vi "doFocus_max-xy.vi"(4 "WFChart Refnum":refnum<vi>, 6 "pixel_dwell_ms":dbl=0.1 caption="Dwell time ms:", 7 "pos_start":enum32{"bottom-left", "center"}(ring), 8 "frame_size_x_px":i32=50, 9 "image_size_x_um":dbl=6.0, 10 "pos-start_y":dbl=6.0, 11 "pos-start_x":dbl=6.0) -> (1 "focus_data":T1, 2 "z-focus":dbl)   [LabVIEW 2014]
panel:
  out "Intensity Graph":dbl[][](graph)
  # "Inputs"
  # "Outputs"
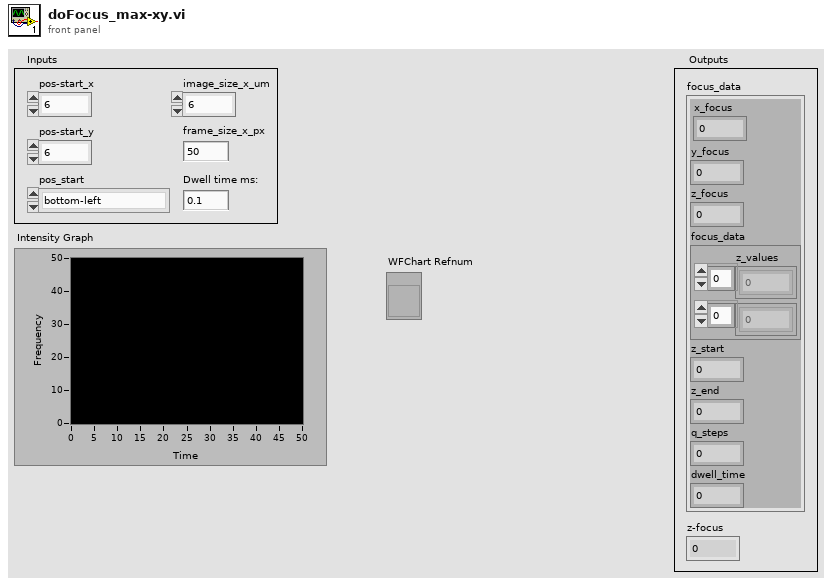
[diagram p1: front panel]
types:
  T1 = cluster{"x_focus":dbl, "y_focus":dbl, "z_focus":dbl, "focus_data":cluster{"z_values":dbl[], dbl[]}, "z_start":dbl, "z_end":dbl, "q_steps":i32, "dwell_time":dbl}
  T2 = cluster{dbl, dbl, "z_focus":dbl, "focus_data":cluster{"z_values":dbl[], dbl[]}, "z_start":dbl, "z_end":dbl, "q_steps":i32, "dwell_time":dbl}
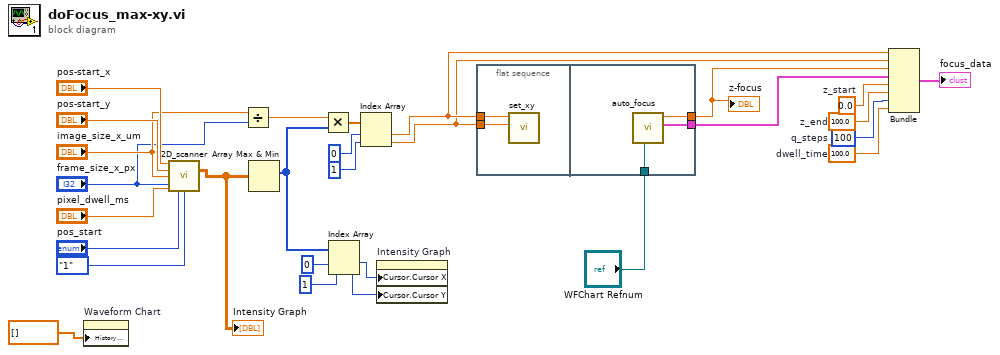
[diagram p0: block diagram]
diagram:
  w3 = 100.0  # dwell_time
  w4 = 100  # q_steps
  w5 = 100.0  # z_end
  w6 = 0.0  # z_start
  n1 = property on="Waveform Chart" class="WFChart (strict)"("History Data"=dbl[] []) -> ()  [unwired: 2 in, 2 out]
  n2 = call "2D_scanner.vi"("pos-start_x"="pos-start_x", "pos-start_y"="pos-start_y", "image_size_x_um"="image_size_x_um", "frame_size_x_px"="frame_size_x_px", "pixel_dwell_ms"="pixel_dwell_ms", "pos_start"="pos_start", "scan_direction"=enum32{"0", "1"}."1") -> ("image_out"=w17:dbl[][])  [unwired: 8 in]
  "Intensity Graph" <- w17
  n3 = Divide(x="image_size_x_um", y="frame_size_x_px") -> (x/y=w22:dbl)
  n4 = Array Max & Min(array=w17) -> (max index (indices)=w16:i32[])  [unwired: 3 out]
  n5 = Multiply(x=w22, y=w16) -> (x*y=w21:dbl[])
  n6 = Index Array(array=w16, index #1=0 ("index"), index #2=1 ("index")) -> (element #1=w13:i32, element #2=w12:i32)
  n7 = Index Array(array=w21, index #1=0 ("index"), index #2=1 ("index")) -> (element #1=w10:dbl, element #2=w9:dbl)
  n8 = property on="Intensity Graph" class="IntGraph (strict)"("Cursor.Cursor X"=w13, "Cursor.Cursor Y"=w12) -> ()  [unwired: 2 in, 2 out]
  n9 = flat-sequence {
    tunnel: w10 -> [w30]
    tunnel: w9 -> [w29]
    tunnel: "WFChart Refnum" -> [w33]
    tunnel: [w32] -> w8
    tunnel: [w31] -> w7
    frame #0 {
      n10 = call "set_xy.vi"("y_value_um"=w29, "x_value_um"=w30) -> ()  [unwired: 9 in, 1 out]
    }
    frame #1 {
      n11 = call "auto_focus.vi"("counts"=w33) -> ("focus_data"=w31:cluster{"z_values":dbl[], dbl[]}, "z_focus"=w32:dbl)  [unwired: 9 in]
    }
  }
  n12 = Bundle(w10, w9, "z_focus"=w8, "focus_data"=w7, "z_start"=w6, "z_end"=w5, "q_steps"=w4, "dwell_time"=w3) -> (→"focus_data":T2)  [unwired: 1 in]
  "z-focus" <- w8
